vi "PDE String Vibration_Init Value.vi"(2 "data":variant, 3 "x":dbl, 4 "t":dbl) -> (0 "error out":errorcluster, 1 "F(t, x)":dbl)   [LabVIEW 2023]
doc: "Generate initial value for PDE String Vibration.vi example."
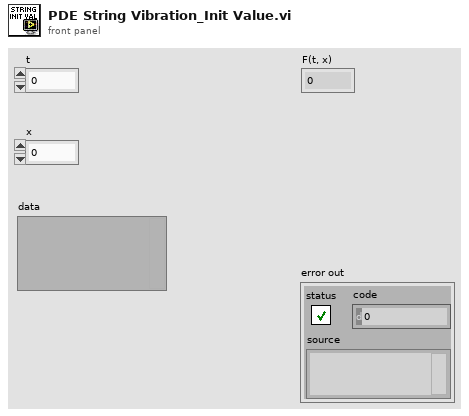
[diagram p1: front panel]
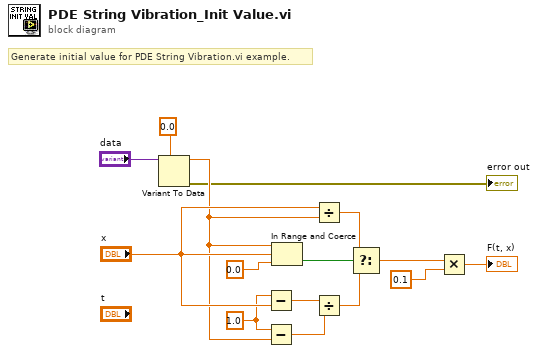
[diagram p0: block diagram]
diagram:
  w1 = 1.0 ("x")
  # "Generate initial value for PDE String Vibration.vi example."
  n1 = Variant To Data(type=0.0, Variant="data") -> (data=w7:dbl, error out=→"error out":errorcluster)  [unwired: 1 in]
  n2 = Subtract(x=w1, y="x") -> (x-y=w11:dbl)
  n3 = Subtract(x=w1, y=w7) -> (x-y=w6:dbl)
  n4 = In Range and Coerce(upper limit=w7, x="x", lower limit=0.0) -> (In Range?=w14:bool)  [unwired: 1 out]
  n5 = Divide(x="x", y=w7) -> (x/y=w12:dbl)
  n6 = Divide(x=w11, y=w6) -> (x/y=w10:dbl)
  n7 = Select(t=w12, s=w14, f=w10) -> (s? t:f=w4:dbl)
  n8 = Multiply(x=w4, y=0.1) -> (x*y=→"F(t, x)":dbl)
